vi "Assign a Vector.vi"(8 "error in":errorcluster, 10 "PVector U in":refnum<class "PVector.lvclass">, 11 "PVector V in":refnum<class "PVector.lvclass">) -> (0 "error out":errorcluster, 3 "PVector V=U out":refnum<class "PVector.lvclass">)   [LabVIEW 2016, in "PVector.lvclass"]
doc: "Perform vector assignment ('=' operation) to make vector V be equivalent to vector U"
uses:
  PVector.lvclass
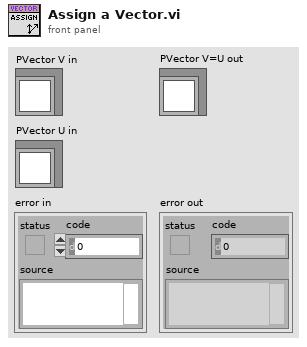
[diagram p1: front panel]
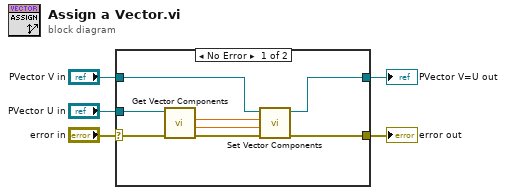
[diagram p0: block diagram]
diagram:
  n1 = case shown="No Error" "error in" {
    selector: "error in" -> [w11 w15]
    tunnel: [w6 w15] -> w4
    tunnel: [w9 w14] -> w2
    tunnel: "PVector V in" -> [w12 w14]
    tunnel: "PVector U in" -> [w13 _]
    frame No Error {
      n2 = call "Get Vector Components.vi"("error in"=w11, "PVector in"=w13) -> ("error out"=w10:errorcluster, "Y"=w7:dbl, "X"=w8:dbl)  [unwired: 6 in, 1 out]
      n3 = call "Set Vector Components.vi"("error in"=w10, "Y"=w7, "X"=w8, "PVector in"=w12) -> ("error out"=w6:errorcluster, "PVector out"=w9:refnum<class "PVector.lvclass">)  [unwired: 6 in]
    }
    frame Error {
    }
  }
  "error out" <- w4
  "PVector V=U out" <- w2
